vi "Write Voltage.vi"(8 "error in":errorcluster, 9 "Channel+Range":string, 10 "Voltage input":i32, 11 "VISA in":refnum<visa-resource-name>) -> (0 "error out":errorcluster, 2 "read buffer":string, 3 "VISA out":refnum<visa-resource-name>)   [LabVIEW 2018]
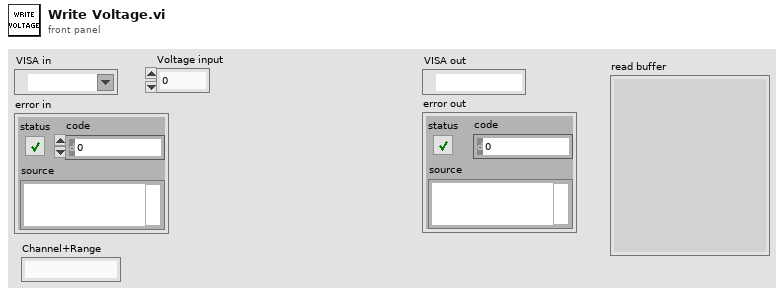
[diagram p1: front panel]
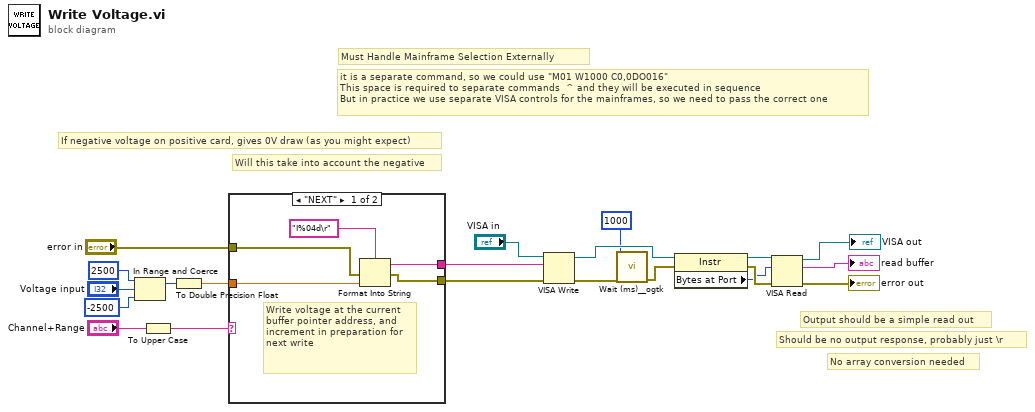
[diagram p0: block diagram]
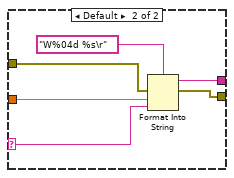
[diagram p2: hidden frame]
diagram:
  # "it is a separate command, so we could use \"M01 W1000 C0,0DO016\"\nThis space is required to separate commands  ^ and they will be executed in sequence\nBut in practice we use separate VISA controls for the mainframes, so we need to pass the correct one"
  # "Must Handle Mainframe Selection Externally"
  # "Should be no output response, probably just \\r"
  # "Will this take into account the negative"
  # "If negative voltage on positive card, gives 0V draw (as you might expect)"
  # "No array conversion needed"
  # "Output should be a simple read out"
  n1 = In Range and Coerce(upper limit=2500, x="Voltage input", lower limit=-2500) -> (coerced(x)=w7:i32)  [unwired: 1 out]
  n2 = To Upper Case(1:"Channel+Range") -> (0:w1:string)
  n3 = To Double Precision Float(number=w7) -> (double precision float=w3:dbl)
  n4 = case shown="\"NEXT\"" w1 {
    selector: w1 -> [_ w28]
    tunnel: [w26 w32] -> w6
    tunnel: "error in" -> [w25 w31]
    tunnel: [w24 w30] -> w4
    tunnel: w3 -> [w23 w29]
    frame "NEXT" {
      # "Write voltage at the current\nbuffer pointer address, and\nincrement in preparation for\nnext write"
      n5 = Format Into String(format string="I%04d\r", error in=w25, w23) -> (resulting string=w26:string, error out=w24:errorcluster)  [unwired: 1 in]
    }
    frame Default {
      n6 = Format Into String(format string="W%04d %s\r", error in=w31, w29, w28) -> (resulting string=w32:string, error out=w30:errorcluster)  [unwired: 1 in]
    }
  }
  n7 = VISA Write(VISA resource name="VISA in", write buffer=w6, error in (no error)=w4) -> (VISA resource name out=w17:refnum<visa-resource-name>, error out=w20:errorcluster)  [unwired: 1 out]
  n8 = call <userlib>:"Wait (ms)__ogtk.vi"("error in (no error)"=w20, "milliseconds to wait"=u32 1000) -> ("error out"=w19:errorcluster)  [unwired: 8 in, 1 out]
  n9 = property class="Instr"(reference=w17, error in=w19) -> (reference out=w15:refnum<visa-resource-name>, error out=w18:errorcluster, "Bytes at Port"=w14:u32)
  n10 = VISA Read(VISA resource name=w15, byte count=w14, error in (no error)=w18) -> (VISA resource name out=→"VISA out":refnum<visa-resource-name>, read buffer=→"read buffer":string, error out=→"error out":errorcluster)  [unwired: 1 out]
